vi "New.vi"(8 "error in (no error)":errorcluster, 10 "timeout":i32=10000, 11 "Socket.TCP in":refnum<class "Socket.TCP.lvclass">) -> (0 "error out":errorcluster, 3 "Socket.TCP out":refnum<class "Socket.TCP.lvclass">)   [LabVIEW 2014, in "Socket.lvlib" / "Socket.TCP.lvclass"]
doc: "socket.New(timeout) creates a new socket object.\n\ni32 timeout network timeout in milliseconds. Default is 10,000 ms (10 seconds)."
uses:
  Socket.TCP.lvclass
  Socket.Base/Socket.Base.lvclass
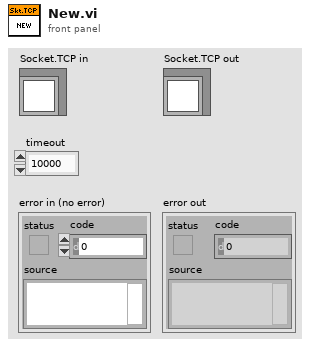
[diagram p1: front panel]
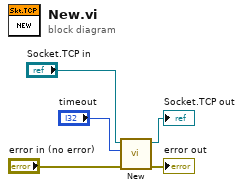
[diagram p0: block diagram]
diagram:
  n1 = call-parent "New.vi"("error in (no error)"="error in (no error)", "timeout"="timeout", "Socket.Base in"="Socket.TCP in") -> ("error out"=→"error out":errorcluster, "Socket.Base out"=→"Socket.TCP out":refnum<class "Socket.TCP.lvclass">)  [unwired: 7 in]
